vi "模式列表删除面板.vi"(9 "pannel ID":i32, 10 "模式":string, 11 "模式列表":T2(array[cluster]) {"sce-pannel-list"."pannel"."ID" format="%02x"}) -> (3 "模式列表 output":T2(array[cluster]) {"sce-pannel-list"."pannel"."ID" format="%02x"})   [LabVIEW 2019]
panel:
  out "模式 2":T1
  out "数组":T2(array[cluster])
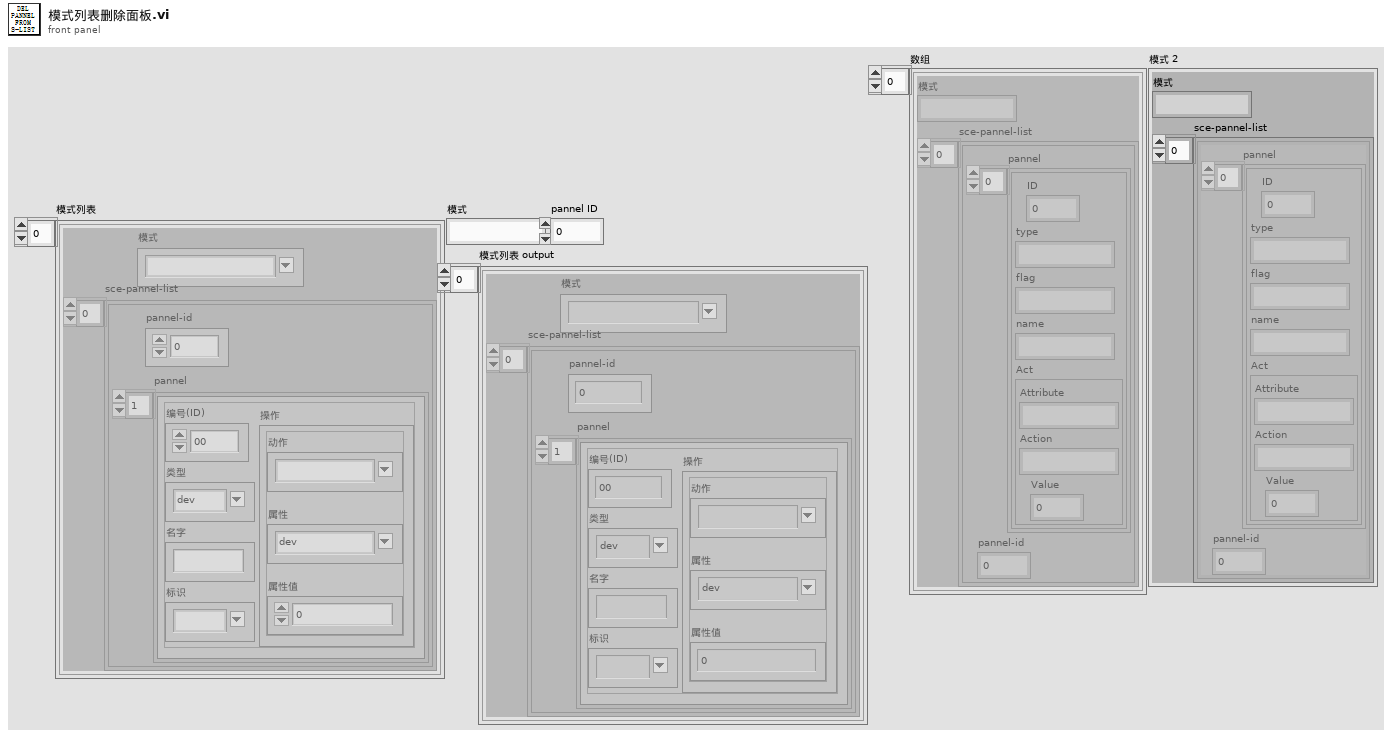
[diagram p1: front panel]
types:
  T1 = cluster{"模式":string, "sce-pannel-list":cluster{"pannel":cluster{"ID":u8, "type":string, "flag":string, "name":string, "Act":cluster{"Attribute":string, "Action":string, "Value":dbl}}[], "pannel-id":dbl}[]}
  T2 = cluster{"模式":string, "sce-pannel-list":cluster{"pannel":cluster{"ID":u8, "type":string, "flag":string, "name":string, "Act":cluster{"Attribute":string, "Action":string, "Value":dbl}}[], "pannel-id":dbl}[]}[]
  T3 = cluster{"pannel":cluster{"ID":u8, "type":string, "flag":string, "name":string, "Act":cluster{"Attribute":string, "Action":string, "Value":dbl}}[], "pannel-id":dbl}[]
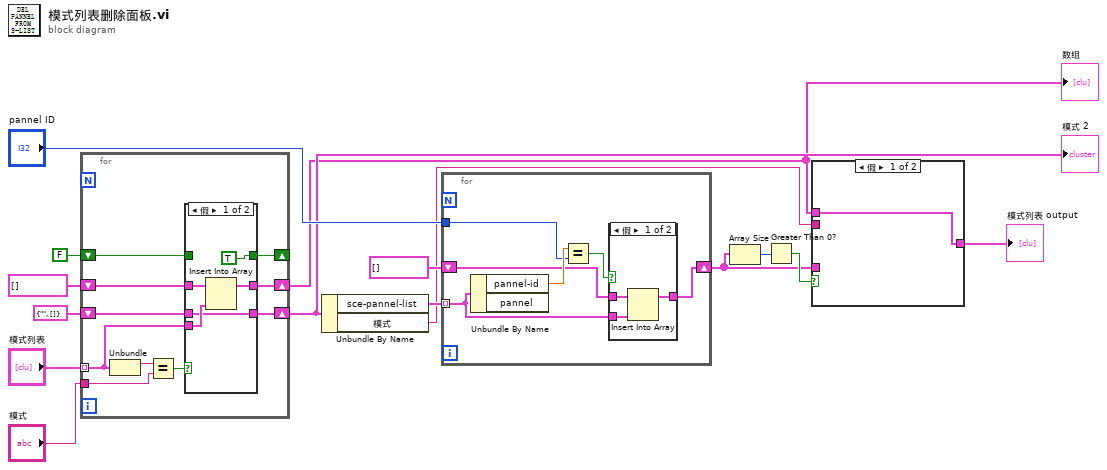
[diagram p0: block diagram]
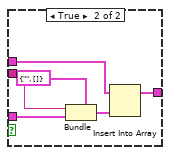
[diagram p2: hidden frame]
diagram:
  n1 = for {
    tunnel: "模式列表" -> [w22] mode=indexing
    tunnel: "模式" -> [w24]
    shift-right: [w21] -> w4
    shift-left: T2 [] -> [w20]
    shift-right: [w19] -> _
    shift-left: FALSE -> [w18]
    shift-right: [w17] -> w5
    shift-left: T1 {"模式"="", "sce-pannel-list"=[]} ("模式 2") -> [w16]
    n2 = Unbundle(w22) -> ("模式"=w25:string)  [unwired: 1 out]
    n3 = Equal?(x=w25, y=w24) -> (x = y?=w23:bool)
    n4 = case shown="假" w23 {
      tunnel: w22 -> [w27 w31]
      tunnel: [w30 w33] -> w21
      tunnel: w20 -> [w29 w33]
      tunnel: [TRUE w32] -> w19
      tunnel: w18 -> [_ w32]
      tunnel: [w26 w31] -> w17
      tunnel: w16 -> [w26 _]
      frame False {
        n5 = Insert Into Array(array=w29, new element=w27) -> (w30:T2)  [unwired: 1 in]
      }
      frame True {
      }
    }
  }
  "数组" <- w4
  "模式 2" <- w5
  n6 = Unbundle By Name(w5) -> ("sce-pannel-list"=w10:T3, "模式"=w2:string)
  n7 = for {
    tunnel: w10 -> [w36] mode=indexing
    shift-right: [w35] -> w3
    shift-left: T3 [] -> [w34]
    tunnel: "pannel ID" -> [w38]
    n8 = Unbundle By Name(w36) -> ("pannel-id"=w39:dbl)  [unwired: 1 out]
    n9 = Equal?(x=w39, y=w38) -> (x = y?=w37:bool)
    n10 = case shown="假" w37 {
      tunnel: w36 -> [w42 _]
      tunnel: [w41 w43] -> w35
      tunnel: w34 -> [w40 w43]
      frame False {
        n11 = Insert Into Array(array=w40, new element=w42) -> (w41:T3)  [unwired: 1 in]
      }
      frame True {
      }
    }
  }
  n12 = Array Size(array=w3) -> (size(s)=w7:i32)
  n13 = Greater Than 0?(x=w7) -> (x > 0?=w6:bool)
  n14 = case shown="假" w6 {
    tunnel: w4 -> [w44 w50]
    tunnel: w3 -> [_ w48]
    tunnel: w2 -> [_ w47]
    tunnel: [w44 w45] -> w1
    frame False {
    }
    frame True {
      n15 = Bundle(cluster=T1 {"模式"="", "sce-pannel-list"=[]} ("模式 2"), "模式"=w47, "sce-pannel-list"=w48) -> (w46:T1)
      n16 = Insert Into Array(array=w50, new element=w46) -> (w45:T2)  [unwired: 1 in]
    }
  }
  "模式列表 output" <- w1
